vi "mqttTCPIPbrokerConnect.vi"(0 "mqtt in":refnum<class "mqtt.lvclass">, 11 "error in (no error)":errorcluster) -> (4 "mqtt out":refnum<class "mqtt.lvclass">, 15 "error out":errorcluster)   [LabVIEW 2017, in "mqtt.lvclass"]
uses:
  mqtt.lvclass
  mqtt.lvclass/mqtt.ctl
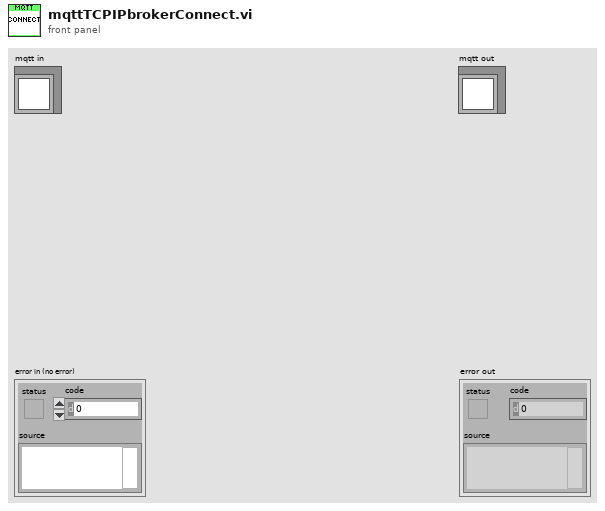
[diagram p1: front panel]
types:
  T1 = typedef "mqttBroker.ctl" = cluster{"address":string, "port":u16, "connTimeout":i32, "writeTimeout":i32, "readTimeout":i32, "subTimeout":i32}
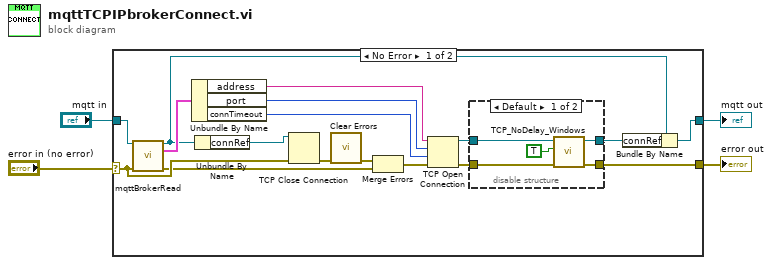
[diagram p0: block diagram]
diagram:
  n1 = case shown="No Error" "error in (no error)" {
    selector: "error in (no error)" -> [w11 w30]
    tunnel: [w5 w30] -> w3
    tunnel: [w14 w29] -> w1
    tunnel: "mqtt in" -> [w16 w29]
    frame No Error {
      n2 = call "mqttBrokerRead.vi"("mqtt in"=w16, "error in (no error)"=w11) -> ("mqtt out"=w13:refnum<class "mqtt.lvclass">, "broker"=w19:T1, "error out"=w8:errorcluster)  [unwired: 11 in]
      n3 = Unbundle By Name(w19) -> ("address"=w18:string, "port"=w17:u16, "connTimeout"=w15:i32)
      n4 = Unbundle By Name(w13) -> ("connRef"=w12:refnum<k5>)
      n5 = TCP Close Connection(connection ID=w12, error in (no error)=w11) -> (error out=w10:errorcluster)  [unwired: 1 in, 1 out]
      n6 = call <vilib>:"Clear Errors.vi"("error in (no error)"=w10) -> ("error out"=w9:errorcluster)  [unwired: 5 in, 1 out]
      n7 = Merge Errors(w9, w8) -> (w7:errorcluster)
      n8 = TCP Open Connection(address=w18, remote port or service name=w17, timeout ms (60000)=w15, error in (no error)=w7) -> (connection ID=w21:refnum<k5>, error out=w20:errorcluster)  [unwired: 1 in]
      n9 = disable-structure shown="Default" {
        disable-tunnel: w21 -> [w26 w28]
        disable-tunnel: w20 -> [w25 w27]
        disable-tunnel: [w24 w27] -> w5
        disable-tunnel: [w22 w28] -> w6
        frame condition #0 (active) {
          n10 = call "TCP_NoDelay_Windows.vi"("error in (no error)"=w25, "TCP_NODELAY (true)"=TRUE, "connID"=w26) -> ("error out"=w24:errorcluster, "connID 2"=w22:refnum<k5>)  [unwired: 3 in]
        }
        frame condition #1 {
        }
      }
      n11 = Bundle By Name(cluster=w13, "connRef"=w6) -> (w14:refnum<class "mqtt.lvclass">)
    }
    frame Error {
    }
  }
  "error out" <- w3
  "mqtt out" <- w1
